vi "midi-tracks.clear.vi"(8 "error in (no error)":errorcluster, 11 "midi-file-events in":refnum<class "midi-file-events.lvclass">) -> (0 "error out":errorcluster, 3 "midi-file-events out":refnum<class "midi-file-events.lvclass">)   [LabVIEW 2020, in "midi-file-events.lvclass"]
uses:
  midi-file-events.lvclass
  midi-file-events.lvclass/midi-file-events.ctl
  midi-file-event/midi-file-event.lvclass
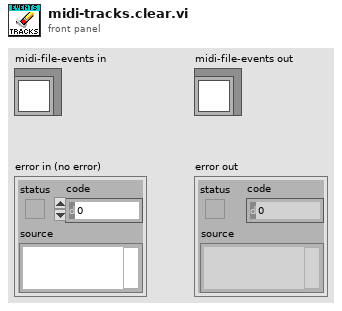
[diagram p1: front panel]
types:
  T1 = map{i32, refnum<class "midi-file-event.lvclass">[]}
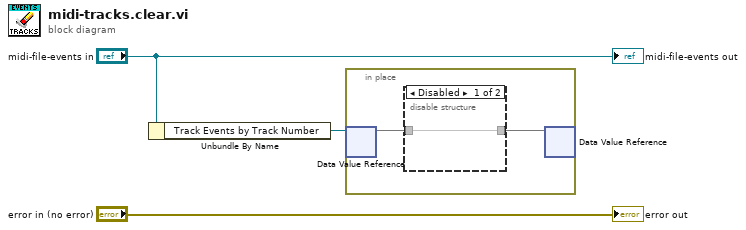
[diagram p0: block diagram]
diagram:
  n1 = Unbundle By Name("midi-file-events in") -> ("Track Events by Track Number"=w3:refnum<data-value>)
  n2 = in-place {
    n3 = in-place-dvr #1(w3) -> (w4:T1)  [unwired: 1 out]
    n4 = disable-structure shown="Disabled" {
      disable-tunnel: [w6 _] -> w5
      disable-tunnel: w4 -> [w6 _]
      frame Disabled {
      }
      frame Enabled {
      }
    }
    n5 = in-place-dvr #1(w5) -> ()  [unwired: 2 out]
  }
  "error out" <- "error in (no error)"
  "midi-file-events out" <- "midi-file-events in"
